vi "OBD_HW_Select.vi"(7 "HW select":u16(ring) items=["NI-XNET", "NI-CAN"], 10 "CAN port":string) -> (2 "CAN port out":string)   [LabVIEW 2018]
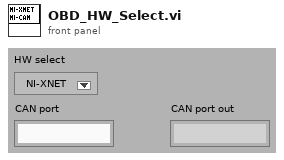
[diagram p1: front panel]
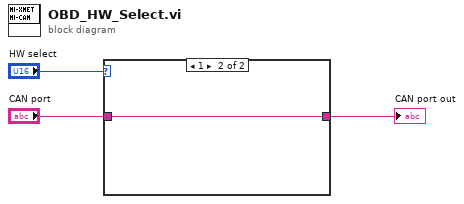
[diagram p0: block diagram]
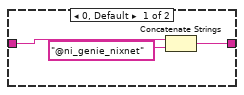
[diagram p2: hidden frame]
diagram:
  n1 = case shown="1" "HW select" {
    tunnel: "CAN port" -> [w6 w7]
    tunnel: [w5 w7] -> w1
    frame 0, Default {
      n2 = Concatenate Strings(w6, "@ni_genie_nixnet" ("string")) -> (w5:string)
    }
    frame 1 {
    }
  }
  "CAN port out" <- w1
